vi "Detect Rotation Direction.vi"(11 "position":u16) -> (2 "previous position (n-1)":u16, 3 "rotated forward or stopped":bool, 5 "cycle wrapped":bool)   [LabVIEW 2013, in "Engine Simulation Toolkit.lvlib"]
uses:
  Engine Simulation Toolkit.lvlib
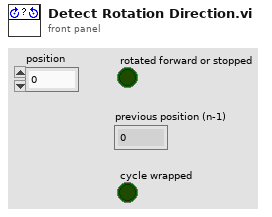
[diagram p1: front panel]
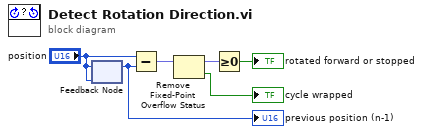
[diagram p0: block diagram]
diagram:
  n1 = feedback #1("position") -> (w5:u16)
  "previous position (n-1)" <- w5
  n2 = feedback-in #1("position") -> ()
  n3 = Subtract(x="position", y=w5) -> (x-y=w4:fxp<+/-,11,11>)
  n4 = Remove Fixed-Point Overflow Status(3:w4) -> (0:→"cycle wrapped":bool, 1:w2:fxp<+/-,11,11>)
  n5 = Greater Or Equal To 0?(x=w2) -> (x >= 0?=→"rotated forward or stopped":bool)
